vi "Custom User Scripting For New Simple Accessor VI.vi"(8 "error in":errorcluster, 10 "Write VI":refnum<vi>, 11 "Read VI":refnum<vi>) -> (0 "error out":errorcluster)   [LabVIEW 2021]
doc: "When \"New >> VI For Data Member Access...\" is used to create VIs, this subVI will be invoked if the VIs are created successfully after all other work to create the VIs has been completed. Users may edit this subVI to add any instructions they wish for customizations of the newly generated VIs."
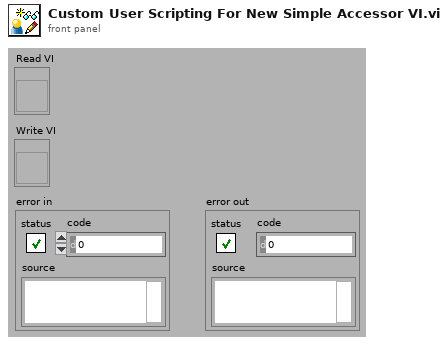
[diagram p1: front panel]
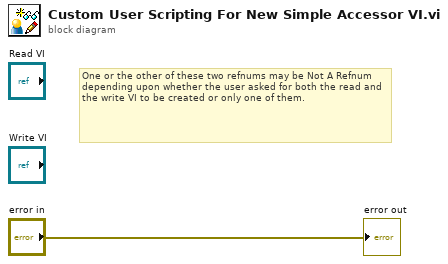
[diagram p0: block diagram]
diagram:
  # "One or the other of these two refnums may be Not A Refnum depending upon whether the user asked for both the read and the write VI to be created or only one of them."
  "error out" <- "error in"
